vi "Restrict X Domain of Graph.vi"(2 "XY Graph":cluster{"Y":dbl[], "Y":dbl[]}[](array[cluster])) -> (0 "Cluster 2":cluster{"Y":dbl[], "Y":dbl[]}, 1 "Cluster":cluster{dbl[], dbl[]})   [LabVIEW 2016]
panel:
  in  "XYGraph Refnum":refnum<vi>
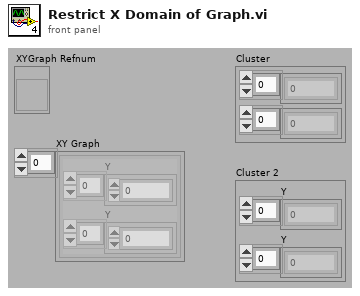
[diagram p1: front panel]
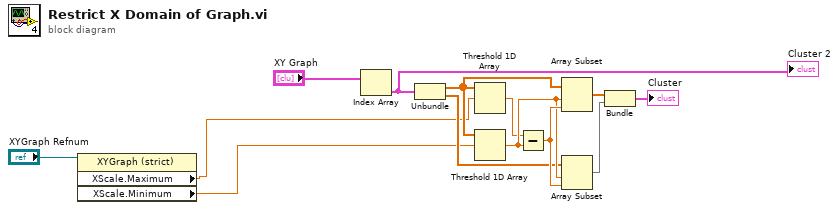
[diagram p0: block diagram]
diagram:
  n1 = property on="Property Node" class="XYGraph (strict)"(reference="XYGraph Refnum") -> ("XScale.Maximum"=w1:dbl, "XScale.Minimum"=w2:dbl)  [unwired: 1 in, 2 out]
  n2 = Index Array(array="XY Graph") -> (element=w5:cluster{"Y":dbl[], "Y":dbl[]})  [unwired: 1 in]
  "Cluster 2" <- w5
  n3 = Unbundle(w5) -> ("Y"=w7:dbl[], "Y"=w8:dbl[])
  n4 = Threshold 1D Array(2:w1, 3:w7) -> (0:w6:dbl)  [unwired: 1 out]
  n5 = Threshold 1D Array(2:w2, 3:w7) -> (0:w9:dbl)  [unwired: 1 out]
  n6 = Subtract(x=w6, y=w9) -> (x-y=w10:dbl)
  n7 = Array Subset(array=w7, index=w9, length=w10) -> (w12:dbl[])
  n8 = Array Subset(array=w8, index=w9, length=w10) -> (w11:dbl[])
  n9 = Bundle(w12, w11) -> (→"Cluster":cluster{dbl[], dbl[]})  [unwired: 1 out]
